vi "Write Active Channel.vi"(8 "error in":errorcluster, 10 "Active Channel":u32, 11 "PowerSupply in":refnum<class "PowerSupply.lvclass">) -> (0 "error out":errorcluster, 3 "PowerSupply out":refnum<class "PowerSupply.lvclass">)   [LabVIEW 2019, in "PowerSupply.lvlib" / "PowerSupply.lvclass"]
uses:
  Library/PowerSupply.lvclass
  C:/Users/Public/Documents/Development/builds/Instruments/Instruments.lvlibp/Library/Instruments.lvclass
  Library/PowerSupply.lvclass/PowerSupply.ctl
  builds/Instruments/Instruments.lvlibp/Accessors/Command with Logging.vi
  builds/Instruments/Instruments.lvlibp/Library/Instruments.lvclass
  builds/Instruments/Instruments.lvlibp/Private/Polymorphic/Special/Event from String.vi
  builds/Instruments/Instruments.lvlibp
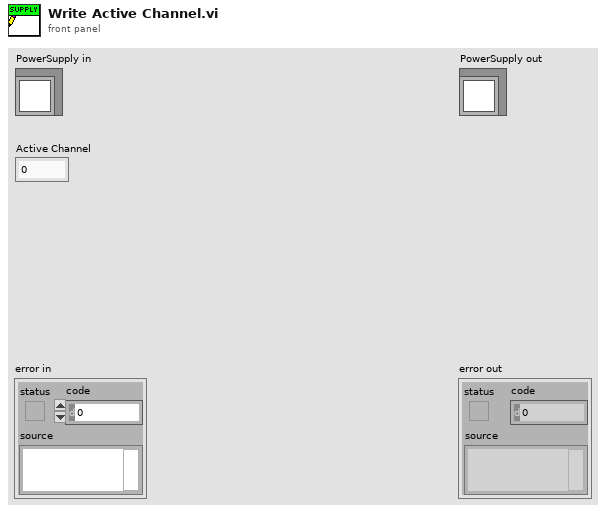
[diagram p1: front panel]
types:
  T1 = cluster{"Timestamp":timestamp, "Description":string, "Data":string}
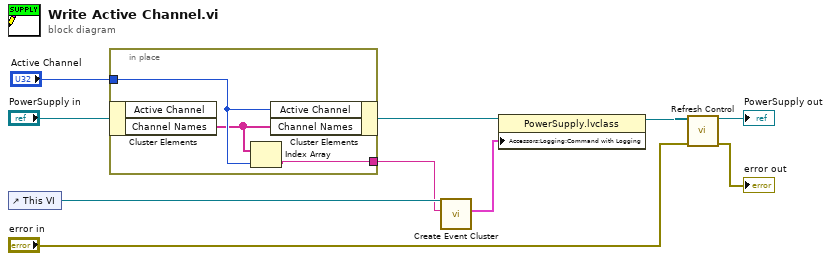
[diagram p0: block diagram]
diagram:
  n1 = control-ref of="This VI"() -> (w7:refnum<vi>)
  n2 = in-place {
    in-place-border: "Active Channel" -> [w13]
    in-place-border: [w11] -> w1
    n3 = in-place-cluster #1("PowerSupply in") -> ("Channel Names"=w12:string[])  [unwired: 1 out]
    n4 = Index Array(array=w12, index=w13) -> (element=w11:string)
    n5 = in-place-cluster #1("Active Channel"=w13, "Channel Names"=w12) -> (w3:refnum<class "PowerSupply.lvclass">)
  }
  n6 = call-poly "Create Event Cluster.vi"("Value"=w1, "VI Refnum"=w7) -> ("Event Data"=w5:T1)  [unwired: 9 in]
  n7 = property class="PowerSupply.lvclass"(reference=w3, "Accessors:Logging:Command with Logging"=w5) -> (reference out=w6:refnum<class "PowerSupply.lvclass">)  [unwired: 1 in, 1 out]
  n8 = call "Refresh Control.vi"("error in"="error in", "PowerSupply in"=w6) -> ("error out"=→"error out":errorcluster, "PowerSupply out"=→"PowerSupply out":refnum<class "PowerSupply.lvclass">)  [unwired: 8 in]
